vi "iWorx Chart Autoscale.vi"(7 "Selection Chart":refnum<vi>, 8 "Error In":errorcluster, 9 "Rounding Multiple (1)":dbl=1.0, 10 "Padding (10%)":dbl=10.0, 11 "Min Range (1)":dbl=1.0) -> (0 "error out":errorcluster, 2 "Min_Rounded":dbl, 3 "Max_Rounded":dbl)   [LabVIEW 2012]
doc: "This subVI is designed to autoscale a waveform chart based on the data that is currently visible on the chart."
uses:
  <vilib>/Utility/miscctls.llb/LVRangeTypeDef.ctl
panel:
  out "Output Scaling":T1
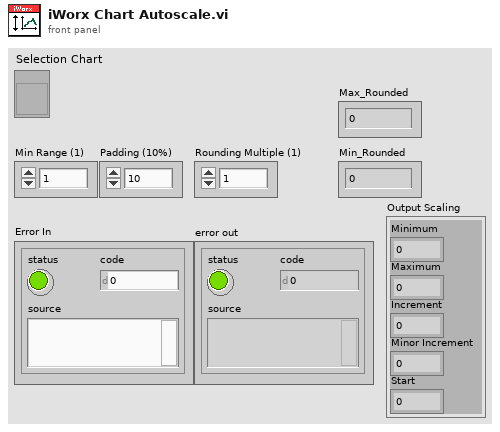
[diagram p1: front panel]
types:
  T1 = typedef "LVRangeTypeDef.ctl" = cluster{"Minimum":dbl, "Maximum":dbl, "Increment":dbl, "Minor Increment":dbl, "Start":dbl}
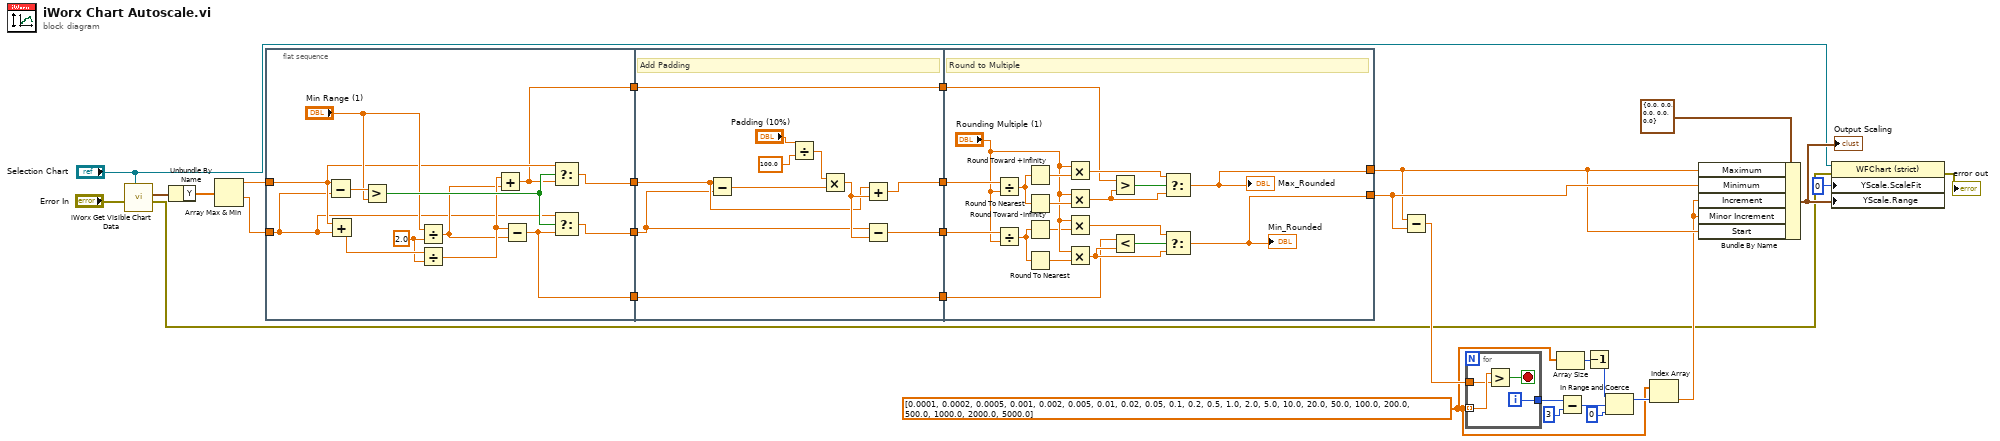
[diagram p0: block diagram]
diagram:
  w8 = dbl[] [0.0001, 0.0002, 0.0005, 0.001, 0.002, 0.005, 0.01, 0.02, 0.05, 0.1, 0.2, 0.5, 1.0, 2.0, 5.0, 10.0, 20.0, 50.0, 100.0, 200.0, 500.0, 1000.0, 2000.0, 5000.0]
  n1 = call "iWorx Get Visible Chart Data.vi"("Selection Chart"="Selection Chart", "error in (no error)"="Error In") -> ("error out"=w3:errorcluster, "waveform out"=w2:waveform(dbl))  [unwired: 7 in, 1 out]
  n2 = Unbundle By Name(w2) -> ("Y"=w18:dbl[])
  n3 = Array Max & Min(array=w18) -> (max value=w31:dbl, min value=w30:dbl)  [unwired: 2 out]
  n4 = flat-sequence {
    tunnel: w30 -> [w33]
    tunnel: w31 -> [w38]
    tunnel: [w37] -> w29
    tunnel: [w36] -> w28
    tunnel: [w35] -> w27
    tunnel: [w34] -> w26
    tunnel: [w48] -> w25
    tunnel: [w47] -> w24
    tunnel: w29 -> [w50]
    tunnel: w28 -> [w49]
    tunnel: [w46] -> w23
    tunnel: w27 -> [w46]
    tunnel: [w45] -> w22
    tunnel: w26 -> [w45]
    tunnel: w25 -> [w74]
    tunnel: w23 -> [w59]
    tunnel: w22 -> [w58]
    tunnel: w24 -> [w73]
    tunnel: [w57] -> w16
    tunnel: [w56] -> w20
    frame #0 {
      w32 = 2.0 ("y")
      n5 = Subtract(x=w38, y=w33) -> (x-y=w44:dbl)
      n6 = Add(x=w38, y=w33) -> (x+y=w42:dbl)
      n7 = Greater?(x=w44, y="Min Range (1)") -> (0:w43:bool)
      n8 = Divide(x="Min Range (1)", y=w32) -> (x/y=w39:dbl)
      n9 = Divide(x=w42, y=w32) -> (x/y=w40:dbl)
      n10 = Add(x=w40, y=w39) -> (x+y=w35:dbl)
      n11 = Subtract(x=w40, y=w39) -> (x-y=w34:dbl)
      n12 = Select(t=w38, s=w43, f=w35) -> (s? t:f=w37:dbl)
      n13 = Select(t=w33, s=w43, f=w34) -> (s? t:f=w36:dbl)
    }
    frame #1 {
      # "Add Padding"
      n14 = Subtract(x=w50, y=w49) -> (x-y=w52:dbl)
      n15 = Divide(x="Padding (10%)", y=100.0) -> (x/y=w53:dbl)
      n16 = Multiply(x=w53, y=w52) -> (x*y=w51:dbl)
      n17 = Add(x=w50, y=w51) -> (x+y=w48:dbl)
      n18 = Subtract(x=w49, y=w51) -> (x-y=w47:dbl)
    }
    frame #2 {
      # "Round to Multiple"
      n19 = Divide(x=w74, y="Rounding Multiple (1)") -> (x/y=w72:dbl)
      n20 = Divide(x=w73, y="Rounding Multiple (1)") -> (x/y=w71:dbl)
      n21 = Round Toward +Infinity(x=w72) -> (ceil(x): smallest int >= x=w68:dbl)
      n22 = Round To Nearest(number=w72) -> (nearest integer value=w67:dbl)
      n23 = Round Toward -Infinity(1:w71) -> (0:w62:dbl)
      n24 = Round To Nearest(number=w71) -> (nearest integer value=w64:dbl)
      n25 = Multiply(x="Rounding Multiple (1)", y=w68) -> (x*y=w66:dbl)
      n26 = Multiply(x="Rounding Multiple (1)", y=w67) -> (x*y=w65:dbl)
      n27 = Multiply(x="Rounding Multiple (1)", y=w62) -> (x*y=w61:dbl)
      n28 = Multiply(x="Rounding Multiple (1)", y=w64) -> (x*y=w60:dbl)
      n29 = Greater?(x=w59, y=w65) -> (0:w70:bool)
      n30 = Less?(x=w58, y=w60) -> (x < y?=w69:bool)
      n31 = Select(t=w66, s=w70, f=w65) -> (s? t:f=w57:dbl)
      "Max_Rounded" <- w57
      n32 = Select(t=w61, s=w69, f=w60) -> (s? t:f=w56:dbl)
      "Min_Rounded" <- w56
    }
  }
  n33 = Subtract(x=w16, y=w20) -> (x-y=w15:dbl)
  n34 = for {
    tunnel: w8 -> [w78] mode=indexing
    tunnel: w15 -> [w77]
    tunnel: [w75] -> w14
    i -> [w75]
    stop <- w76 stop-if-true
    n35 = Greater?(x=w78, y=w77) -> (0:w76:bool)
  }
  n36 = Array Size(array=w8) -> (size(s)=w7:i32)
  n37 = Subtract(x=w14, y=3 ("x")) -> (x-y=w11:i32)
  n38 = Decrement(x=w7) -> (x-1=w6:i32)
  n39 = In Range and Coerce(upper limit=w6, x=w11, lower limit=0) -> (coerced(x)=w9:i32)  [unwired: 1 out]
  n40 = Index Array(array=w8, index=w9) -> (element=w13:dbl)
  n41 = Bundle By Name(cluster=T1 {"Minimum"=0.0, "Maximum"=0.0, "Increment"=0.0, "Minor Increment"=0.0, "Start"=0.0} ("Y Scale.Range"), "Maximum"=w16, "Minimum"=w20, "Increment"=w13, "Minor Increment"=w13, "Start"=w16) -> (w19:T1)
  "Output Scaling" <- w19
  n42 = property class="WFChart (strict)"(reference="Selection Chart", error in=w3, "YScale.ScaleFit"=u8 0 ("Y Scale.Scale Fit"), "YScale.Range"=w19) -> (error out=→"error out":errorcluster)  [unwired: 1 out]
